vi "Read Config.vi"(8 "error in (no error)":errorcluster) -> (0 "error out":errorcluster, 3 "value":T1)   [LabVIEW 2020, in "Monedas.lvlib"]
uses:
  Monedas.lvlib
  Type defMonedasread.ctl
  <vilib>/Utility/xml.llb/Read From XML File(string).vi
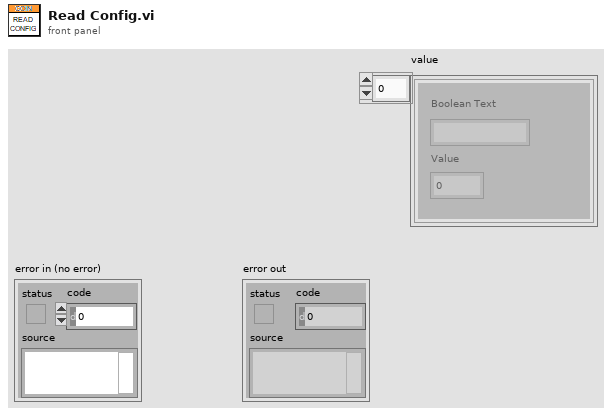
[diagram p1: front panel]
types:
  T1 = typedef "Type defMonedasread.ctl" = cluster{"Boolean Text":string, "Value":dbl}[]
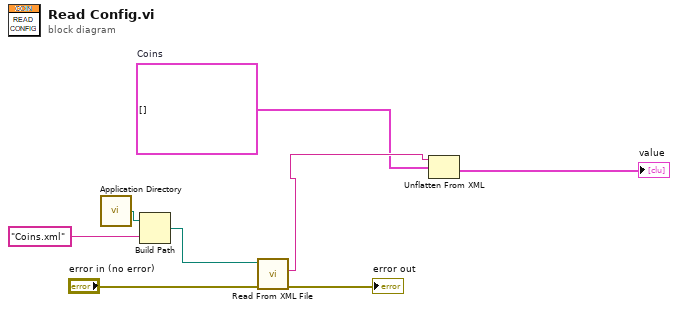
[diagram p0: block diagram]
diagram:
  w1 = cluster{"Boolean Text":string, "Value":dbl}[] []  # Coins
  n1 = call <vilib>:"Application Directory.vi"() -> ("Application Directory"=w8:path)
  n2 = Build Path(base path=w8, name or relative path="Coins.xml") -> (appended path=w4:path)
  n3 = call-poly <vilib>:"Read From XML File.vi"("error in (no error)"="error in (no error)", "XML File Path"=w4) -> ("error out"=→"error out":errorcluster, "XML Elements"=w2:string)  [unwired: 7 in, 1 out]
  n4 = Unflatten From XML(xml string=w2, type=w1) -> (value=→"value":cluster{"Boolean Text":string, "Value":dbl}[])  [unwired: 1 in, 1 out]
